vi "Three part faster sub.vi"() -> ()   [LabVIEW 2009]
uses:
  <vilib>/vision/Image Controls.llb/IMAQ Image.ctl
  <vilib>/Instr/_visa.llb/VISA Configure Serial Port (Instr).vi
  <vilib>/vision/NI_Vision_Development_Module.lvlib
panel:
  in  "VISA resource name":refnum<visa-resource-name>
  out "number":u8 format="%b"
  out "decimal integer string":string
  out "decimal integer string 2":string
  out "decimal integer string 3":string
  out "number 2":u8 format="%b"
  out "number 3":u8 format="%b"
  out "Guitar Cluster":T1
  out "Bass Cluster":T2
  out "Drum Cluster":T3
  out "Image 2":T4(plugin-control)
  in  "Orange Bass":T5={"Global Rectangle"=[220, 302, 227, 392], "Contours"=[{"ID"=enum."External", "Type"=2, "Coordinates"=[226, 391, 220, 302]}]} {"Contours"."Type" items=["No Selection", "Point", "Line", "Rectangle", "Oval", "Polygon", "Freehand Region", "Annulus", "Unused2", "Unused3", "Broken Line", "Freehand Line", "Rotated Rectangle"]}
  in  "Blue Bass":T5={"Global Rectangle"=[192, 292, 199, 386], "Contours"=[{"ID"=enum."External", "Type"=2, "Coordinates"=[192, 385, 198, 292]}]} {"Contours"."Type" items=["No Selection", "Point", "Line", "Rectangle", "Oval", "Polygon", "Freehand Region", "Annulus", "Unused2", "Unused3", "Broken Line", "Freehand Line", "Rotated Rectangle"]}
  in  "playtime":dbl=30.0
  in  "Orange Guitar":T5={"Global Rectangle"=[587, 282, 628, 378], "Contours"=[{"ID"=enum."External", "Type"=2, "Coordinates"=[627, 377, 587, 282]}]} {"Contours"."Type" items=["No Selection", "Point", "Line", "Rectangle", "Oval", "Polygon", "Freehand Region", "Annulus", "Unused2", "Unused3", "Broken Line", "Freehand Line", "Rotated Rectangle"]}
  in  "Yellow Guitar":T5={"Global Rectangle"=[546, 282, 563, 376], "Contours"=[{"ID"=enum."External", "Type"=2, "Coordinates"=[562, 375, 546, 282]}]} {"Contours"."Type" items=["No Selection", "Point", "Line", "Rectangle", "Oval", "Polygon", "Freehand Region", "Annulus", "Unused2", "Unused3", "Broken Line", "Freehand Line", "Rotated Rectangle"]}
  in  "Green Guitar":T5={"Global Rectangle"=[498, 284, 505, 376], "Contours"=[{"ID"=enum."External", "Type"=2, "Coordinates"=[498, 375, 504, 284]}]} {"Contours"."Type" items=["No Selection", "Point", "Line", "Rectangle", "Oval", "Polygon", "Freehand Region", "Annulus", "Unused2", "Unused3", "Broken Line", "Freehand Line", "Rotated Rectangle"]}
  in  "Blue Guitar":T5={"Global Rectangle"=[569, 290, 594, 372], "Contours"=[{"ID"=enum."External", "Type"=2, "Coordinates"=[593, 371, 569, 290]}]} {"Contours"."Type" items=["No Selection", "Point", "Line", "Rectangle", "Oval", "Polygon", "Freehand Region", "Annulus", "Unused2", "Unused3", "Broken Line", "Freehand Line", "Rotated Rectangle"]}
  in  "Red Guitar":T5={"Global Rectangle"=[526, 284, 530, 370], "Contours"=[{"ID"=enum."External", "Type"=2, "Coordinates"=[529, 369, 526, 284]}]} {"Contours"."Type" items=["No Selection", "Point", "Line", "Rectangle", "Oval", "Polygon", "Freehand Region", "Annulus", "Unused2", "Unused3", "Broken Line", "Freehand Line", "Rotated Rectangle"]}
  in  "Green Bass":T5={"Global Rectangle"=[100, 292, 131, 371], "Contours"=[{"ID"=enum."External", "Type"=2, "Coordinates"=[100, 370, 130, 292]}]} {"Contours"."Type" items=["No Selection", "Point", "Line", "Rectangle", "Oval", "Polygon", "Freehand Region", "Annulus", "Unused2", "Unused3", "Broken Line", "Freehand Line", "Rotated Rectangle"]}
  in  "Red Bass":T5={"Global Rectangle"=[129, 294, 154, 376], "Contours"=[{"ID"=enum."External", "Type"=2, "Coordinates"=[129, 375, 153, 294]}]} {"Contours"."Type" items=["No Selection", "Point", "Line", "Rectangle", "Oval", "Polygon", "Freehand Region", "Annulus", "Unused2", "Unused3", "Broken Line", "Freehand Line", "Rotated Rectangle"]}
  in  "Yellow Bass":T5={"Global Rectangle"=[160, 295, 175, 378], "Contours"=[{"ID"=enum."External", "Type"=2, "Coordinates"=[160, 377, 174, 295]}]} {"Contours"."Type" items=["No Selection", "Point", "Line", "Rectangle", "Oval", "Polygon", "Freehand Region", "Annulus", "Unused2", "Unused3", "Broken Line", "Freehand Line", "Rotated Rectangle"]}
  in  "Mask":T5 {"Contours"."Type" items=["No Selection", "Point", "Line", "Rectangle", "Oval", "Polygon", "Freehand Region", "Annulus", "Unused2", "Unused3", "Broken Line", "Freehand Line", "Rotated Rectangle"]}
  in  "Red Line":T5={"Global Rectangle"=[300, 297, 320, 380], "Contours"=[{"ID"=enum."External", "Type"=2, "Coordinates"=[300, 379, 319, 297]}]} {"Contours"."Type" items=["No Selection", "Point", "Line", "Rectangle", "Oval", "Polygon", "Freehand Region", "Annulus", "Unused2", "Unused3", "Broken Line", "Freehand Line", "Rotated Rectangle"]}
  in  "Blue Line":T5={"Global Rectangle"=[374, 278, 383, 377], "Contours"=[{"ID"=enum."External", "Type"=2, "Coordinates"=[382, 376, 374, 278]}]} {"Contours"."Type" items=["No Selection", "Point", "Line", "Rectangle", "Oval", "Polygon", "Freehand Region", "Annulus", "Unused2", "Unused3", "Broken Line", "Freehand Line", "Rotated Rectangle"]}
  in  "Green Line":T5={"Global Rectangle"=[406, 309, 423, 383], "Contours"=[{"ID"=enum."External", "Type"=2, "Coordinates"=[422, 382, 406, 309]}]} {"Contours"."Type" items=["No Selection", "Point", "Line", "Rectangle", "Oval", "Polygon", "Freehand Region", "Annulus", "Unused2", "Unused3", "Broken Line", "Freehand Line", "Rotated Rectangle"]}
  in  "Yellow Line":T5={"Global Rectangle"=[342, 292, 349, 377], "Contours"=[{"ID"=enum."External", "Type"=2, "Coordinates"=[342, 376, 348, 292]}]} {"Contours"."Type" items=["No Selection", "Point", "Line", "Rectangle", "Oval", "Polygon", "Freehand Region", "Annulus", "Unused2", "Unused3", "Broken Line", "Freehand Line", "Rotated Rectangle"]}
  out "Image Dst Out":T4
  out "Frame Number":i32
  in  "Frame Start":i32
  in  "stop":bool
  in  "AVI Path":path
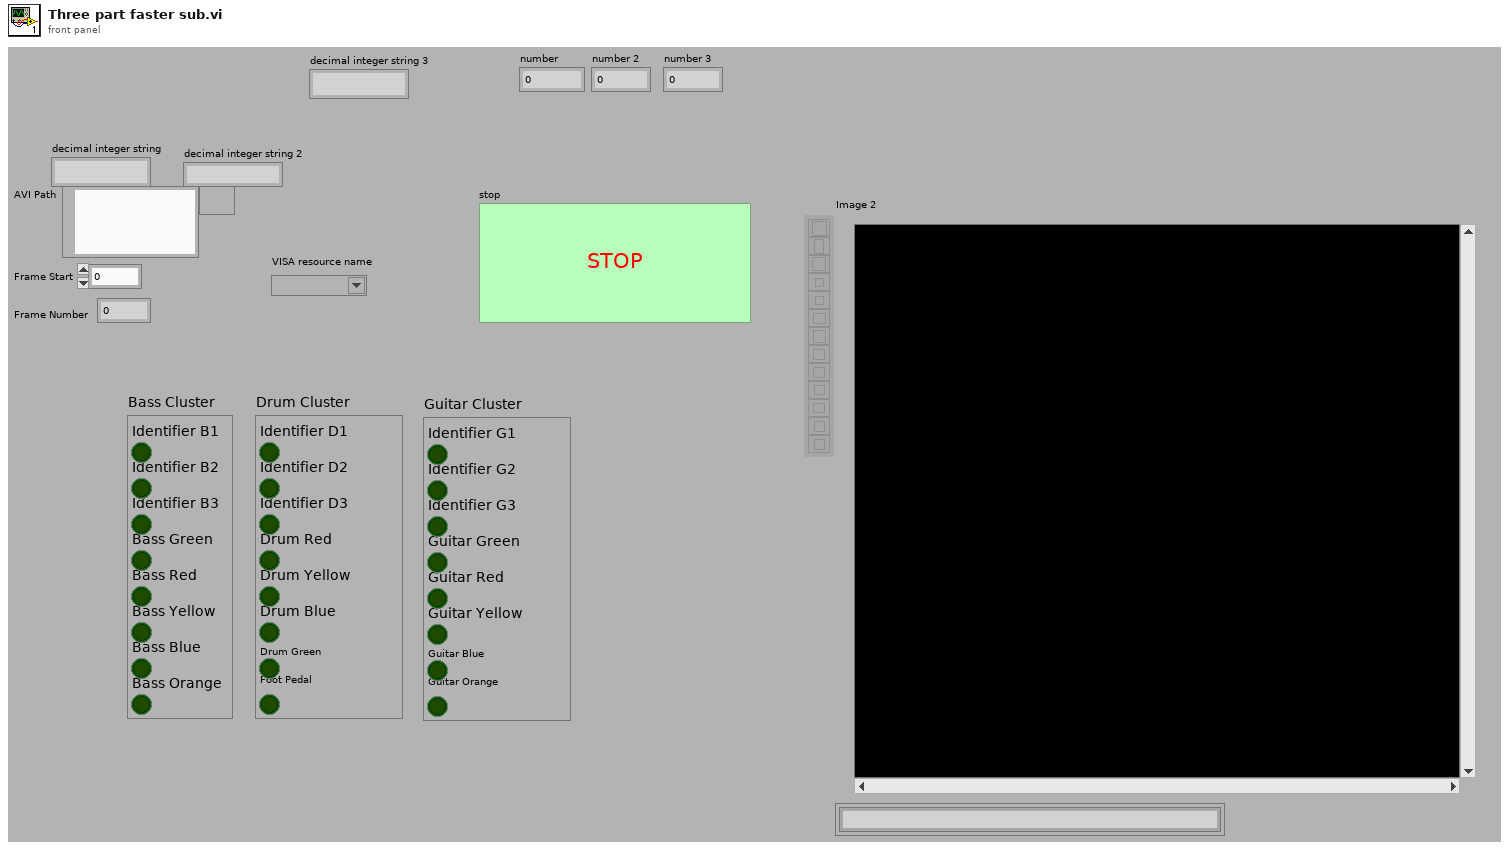
[diagram p1: front panel]
types:
  T1 = cluster{"Identifier G1":bool, "Identifier G2":bool, "Identifier G3":bool, "Guitar Green":bool, "Guitar Red":bool, "Guitar Yellow":bool, "Guitar Blue":bool, "Guitar Orange":bool}
  T2 = cluster{"Identifier B1":bool, "Identifier B2":bool, "Identifier B3":bool, "Bass Green":bool, "Bass Red":bool, "Bass Yellow":bool, "Bass Blue ":bool, "Bass Orange":bool}
  T3 = cluster{"Identifier D1":bool, "Identifier D2":bool, "Identifier D3":bool, "Drum Red":bool, "Drum Yellow":bool, "Drum Blue":bool, "Drum Green":bool, "Foot Pedal":bool}
  T4 = typedef "IMAQ Image.ctl" = refnum<image>
  T5 = cluster{"Global Rectangle":i32[], "Contours":cluster{"ID":enum32{"External", "Internal"}, "Type":u32, "Coordinates":i32[]}[]}
  T6 = typedef "Image Type" = u32
  T7 = typedef "AviRefnum.ctl" = refnum<k1>
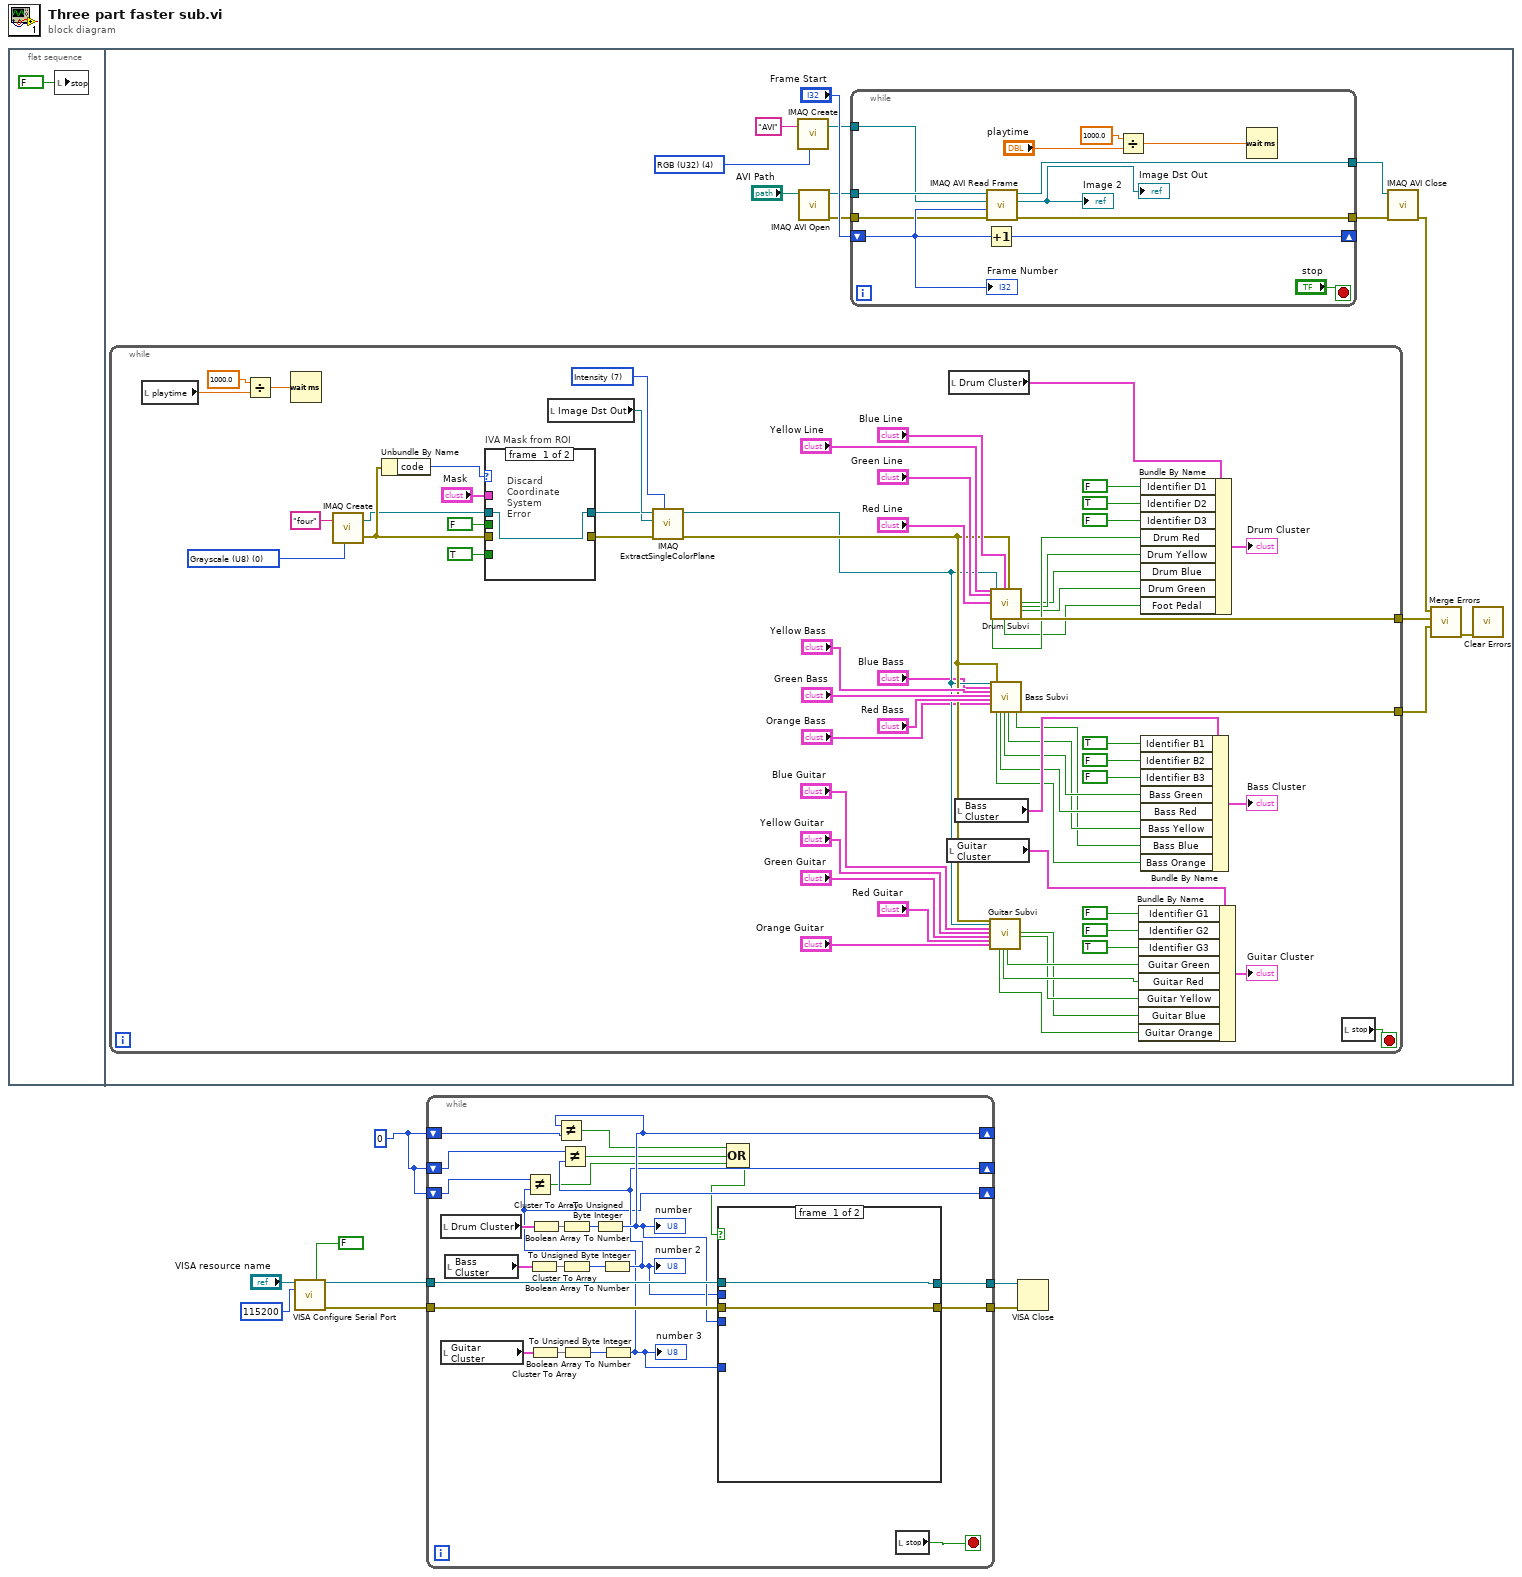
[diagram p0: block diagram]
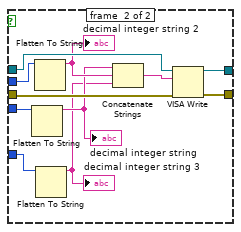
[diagram p2: hidden frame]
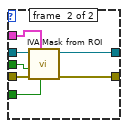
[diagram p3: hidden frame]
diagram:
  w1 = u8 0
  n1 = flat-sequence {
    frame #0 {
      n2 = local write "stop"(FALSE ("stop")) -> ()
    }
    frame #1 {
      w14 = T6 4 items=["Grayscale (U8)", "Grayscale (I16)", "Grayscale (SGL)", "Complex (CSG)", "RGB (U32)", "HSL (U32)", "RGB (U64)", "Grayscale (U16)"] ("Image Type")
      n3 = while {
        tunnel: [w71] -> w11
        tunnel: [w63] -> w10
        stop <- w85 stop-if-true
        w81 = T6 0 items=["Grayscale (U8)", "Grayscale (I16)", "Grayscale (SGL)", "Complex (CSG)", "RGB (U32)", "HSL (U32)", "RGB (U64)", "Grayscale (U16)"] ("Image Type")
        w86 = 7 items=["Red", "Green", "Blue", "Hue", "Saturation", "Luminance", "Value", "Intensity"] ("Color Plane")
        n4 = local read "playtime"() -> (w55:dbl)
        n5 = Divide(x=1000.0, y=w55) -> (x/y=w84:dbl)
        n6 = Wait (ms)(milliseconds to wait=w84) -> ()  [unwired: 1 out]
        n7 = call "IMAQ Create"("Image Name"="four", "Image Type"=w81) -> ("New Image"=w74:T4, "error out"=w75:errorcluster)  [unwired: 3 in]
        n8 = Unbundle By Name(w75) -> ("code"=w79:i32)
        n9 = case "IVA Mask from ROI" shown="Default" w79 {
          tunnel: "Mask" -> [_ w94]
          tunnel: TRUE ("Shrink") -> [_ w93]
          tunnel: w74 -> [w87 w92]
          tunnel: w75 -> [_ w91]
          tunnel: [_ w90] -> w76
          tunnel: [w87 w89] -> w72
          tunnel: FALSE ("Out / In") -> [_ w88]
          frame #0 {
            # "Discard\nCoordinate\nSystem\nError"
          }
          frame #1 {
            n10 = call <vilib>:"IVA Mask from ROI.vi"("Shrink"=w93, "ROI Descriptor"=w94, "error in (no error)"=w91, "Out / In"=w88, "Image Src"=w92) -> ("error out"=w90:errorcluster, "Image Out"=w89:T4)  [unwired: 5 out]
          }
        }
        n11 = local read "Image Dst Out"() -> (w82:T4)
        n12 = call "IMAQ ExtractSingleColorPlane"("Color Plane"=w86, "error in (no error)"=w76, "Image Dst"=w72, "Image Src"=w82) -> ("error out"=w62:errorcluster, "Image Dst Out"=w57:T4)  [unwired: 6 out]
        n13 = local read "Guitar Cluster"() -> (w31:T1)
        n14 = local read "Drum Cluster"() -> (w51:T3)
        n15 = local read "Bass Cluster"() -> (w42:T2)
        n16 = call "Guitar Subvi.vi"("error out"=w62, "Image Dst Out"=w57, "Blue Guitar 2"="Blue Guitar", "Yellow Guitar 2"="Yellow Guitar", "Green Guitar 2"="Green Guitar", "Red Guitar 2"="Red Guitar", "Orange Guitar 2"="Orange Guitar") -> ("Orange Guitar LED"=w23:bool, "Red Guitar LED"=w26:bool, "Green Guitar LED"=w27:bool, "Blue Guitar LED"=w24:bool, "Yellow Guitar LED"=w25:bool)  [unwired: 16 in]
        n17 = call "Drum Subvi.vi"("Yellow Line"="Yellow Line", "Green Line"="Green Line", "Red Line"="Red Line", "Image Dst Out"=w57, "Blue Line"="Blue Line", "error out"=w62) -> ("LED Red"=w50:bool, "Foot Pedal"=w46:bool, "Blue Drum 2"=w48:bool, "Yellow Drum"=w49:bool, "Green Drum"=w47:bool, "error out 2"=w71:errorcluster)  [unwired: 12 in, 4 out]
        n18 = call "Bass Subvi.vi"("Image Dst Out"=w57, "Blue Bass 2"="Blue Bass", "Yellow Bass 2"="Yellow Bass", "Green Bass 2"="Green Bass", "Red Bass 2"="Red Bass", "Orange Bass 2"="Orange Bass", "error out"=w62) -> ("Orange Bass LED"=w33:bool, "Red Bass LED"=w36:bool, "Green Bass LED"=w37:bool, "Yellow Bass LED"=w35:bool, "Blue Bass LED"=w34:bool, "error out 2"=w63:errorcluster)  [unwired: 15 in]
        n19 = Bundle By Name(cluster=w31, "Identifier G1"=FALSE ("element"), "Identifier G2"=FALSE ("element"), "Identifier G3"=TRUE ("element"), "Guitar Green"=w27, "Guitar Red"=w26, "Guitar Yellow"=w25, "Guitar Blue"=w24, "Guitar Orange"=w23) -> (→"Guitar Cluster":T1)
        n20 = Bundle By Name(cluster=w51, "Identifier D1"=FALSE ("D1"), "Identifier D2"=TRUE ("D2"), "Identifier D3"=FALSE ("D3"), "Drum Red"=w50, "Drum Yellow"=w49, "Drum Blue"=w48, "Drum Green"=w47, "Foot Pedal"=w46) -> (→"Drum Cluster":T3)
        n21 = Bundle By Name(cluster=w42, "Identifier B1"=TRUE, "Identifier B2"=FALSE ("element"), "Identifier B3"=FALSE ("element"), "Bass Green"=w37, "Bass Red"=w36, "Bass Yellow"=w35, "Bass Blue"=w34, "Bass Orange"=w33) -> (→"Bass Cluster":T2)
        n22 = local read "stop"() -> (w85:bool)
      }
      n23 = call "IMAQ Create"("Image Name"="AVI", "Image Type"=w14) -> ("New Image"=w12:T4)  [unwired: 3 in, 1 out]
      n24 = call "IMAQ AVI Open"("AVI Path"="AVI Path") -> ("error out"=w19:errorcluster, "Avi Refnum"=w20:T7)  [unwired: 9 in]
      n25 = while {
        tunnel: w20 -> [w106]
        tunnel: w19 -> [w98]
        tunnel: [w105] -> w21
        shift-right: [w100] -> _
        shift-left: "Frame Start" -> [w99]
        tunnel: [w97] -> w15
        tunnel: w12 -> [w96]
        stop <- "stop" stop-if-true
        n26 = Increment(x=w99) -> (x+1=w100:i32)
        n27 = call "IMAQ AVI Read Frame"("error in (no error)"=w98, "Frame Number"=w99, "Image"=w96, "Avi Refnum"=w106) -> ("error out"=w97:errorcluster, "Image Out"=→"Image Dst Out" →"Image 2":T4, "Avi Refnum (duplicate)"=w105:T7)  [unwired: 4 in, 1 out]
        n28 = Divide(x=1000.0, y="playtime") -> (x/y=w103:dbl)
        n29 = Wait (ms)(milliseconds to wait=w103) -> ()  [unwired: 1 out]
        "Frame Number" <- w99
      }
      n30 = call "IMAQ AVI Close"("error in (no error)"=w15, "Avi Refnum"=w21) -> ("error out"=w17:errorcluster)  [unwired: 9 in]
      n31 = call <vilib>:"Merge Errors.vi"("error in 3 (no error)"=w10, "error in 2 (no error)"=w11, "error in 1 (no error)"=w17) -> ("error out"=w16:errorcluster)  [unwired: 4 in]
      n32 = call <vilib>:"Clear Errors.vi"("error in (no error)"=w16) -> ()  [unwired: 6 in, 1 out]
    }
  }
  n33 = call-poly "VISA Configure Serial Port"("VISA resource name"="VISA resource name", "Enable Termination\nChar (T)"=FALSE ("Enable Termination\nChar (T)"), "baud rate (9600)"=u32 115200) -> ("VISA resource name out"=w8:refnum<visa-resource-name>, "error out"=w3:errorcluster)  [unwired: 11 in]
  n34 = while {
    tunnel: w8 -> [w130]
    tunnel: [w129] -> w7
    tunnel: w3 -> [w128]
    tunnel: [w127] -> w2
    shift-right: [w119] -> _
    shift-left: w1 -> [w118]
    shift-right: [w117] -> _
    shift-left: w1 -> [w116]
    shift-right: [w111] -> _
    shift-left: w1 -> [w112]
    stop <- w122 stop-if-true
    n35 = local read "Drum Cluster"() -> (w123:T3)
    n36 = local read "Guitar Cluster"() -> (w114:T1)
    n37 = local read "Bass Cluster"() -> (w124:T2)
    n38 = Cluster To Array(cluster=w124) -> (array=w125:bool[])
    n39 = Cluster To Array(cluster=w114) -> (array=w113:bool[])
    n40 = Cluster To Array(cluster=w123) -> (array=w126:bool[])
    n41 = Boolean Array To Number(Boolean array=w126) -> (number=w121:u32)
    n42 = Boolean Array To Number(Boolean array=w125) -> (number=w120:u32)
    n43 = Boolean Array To Number(Boolean array=w113) -> (number=w115:u32)
    n44 = To Unsigned Byte Integer(number=w121) -> (unsigned 8bit integer=w119:u8)
    "number" <- w119
    n45 = Not Equal?(x=w119, y=w118) -> (x != y?=w109:bool)
    n46 = To Unsigned Byte Integer(number=w120) -> (unsigned 8bit integer=w117:u8)
    "number 2" <- w117
    n47 = Not Equal?(x=w116, y=w117) -> (x != y?=w108:bool)
    n48 = To Unsigned Byte Integer(number=w115) -> (unsigned 8bit integer=w111:u8)
    "number 3" <- w111
    n49 = Not Equal?(x=w112, y=w111) -> (x != y?=w107:bool)
    n50 = Compound Arithmetic op=OR(w109, w108, w107) -> (w110:bool)
    n51 = case shown="True" w110 {
      tunnel: w130 -> [w132 w143]
      tunnel: [w132 w142] -> w129
      tunnel: w119 -> [_ w136]
      tunnel: w128 -> [w131 w141]
      tunnel: [w131 w140] -> w127
      tunnel: w117 -> [_ w138]
      tunnel: w111 -> [_ w133]
      frame #0 {
      }
      frame #1 {
        n52 = Flatten To String(anything=w136) -> (data string=w135:string)  [unwired: 3 in, 2 out]
        "decimal integer string" <- w135
        n53 = Flatten To String(anything=w138) -> (data string=w137:string)  [unwired: 3 in, 2 out]
        "decimal integer string 2" <- w137
        n54 = Flatten To String(anything=w133) -> (data string=w134:string)  [unwired: 3 in, 2 out]
        "decimal integer string 3" <- w134
        n55 = Concatenate Strings(w135, w137, w134) -> (w139:string)
        n56 = VISA Write(VISA resource name=w143, write buffer=w139, error in (no error)=w141) -> (VISA resource name out=w142:refnum<visa-resource-name>, error out=w140:errorcluster)  [unwired: 1 out]
      }
    }
    n57 = local read "stop"() -> (w122:bool)
  }
  n58 = VISA Close(VISA resource name=w7, error in (no error)=w2) -> ()  [unwired: 1 out]
